vi "get_endpoint.vi"(8 "error in (no error)":errorcluster, 11 "WebSocket Connection in":refnum<class "WebSocket Connection.lvclass">) -> (0 "error out":errorcluster, 1 "remote port":u16, 2 "remote address":string, 3 "WebSocket Connection out":refnum<class "WebSocket Connection.lvclass">)   [LabVIEW 2019, in "WebSocket Server Toolkit.lvlib" / "WebSocket Connection.lvclass"]
uses:
  WebSocket Connection.lvclass
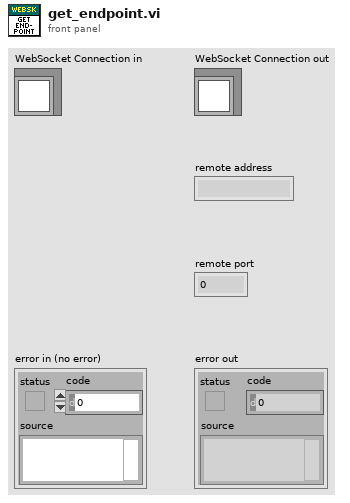
[diagram p1: front panel]
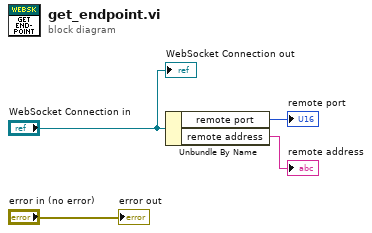
[diagram p0: block diagram]
diagram:
  n1 = Unbundle By Name("WebSocket Connection in") -> ("remote port"=→"remote port":u16, "remote address"=→"remote address":string)
  "error out" <- "error in (no error)"
  "WebSocket Connection out" <- "WebSocket Connection in"
